vi "Example 02e - Lua Scripts from Lua File.vi"() -> ()   [LabVIEW 2020]
uses:
  Lua for LabVIEW/Lua/Lua.lvclass
panel:
  out "-number":dbl
  out "-integer":i64
  out "!boolean":bool
  out "upper(string)":string
  in  "an_integer":i64=58812
  in  "a boolean":bool=TRUE
  in  "a string":string="my name is ..."
  in  "a double":dbl=2.2
  out "error out":errorcluster
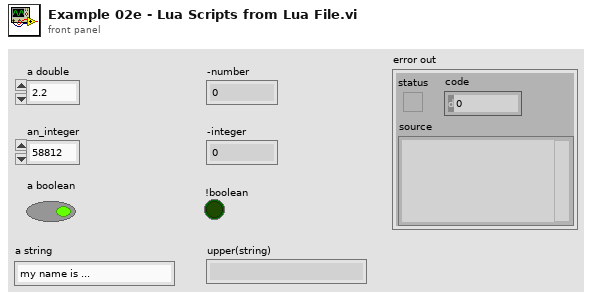
[diagram p1: front panel]
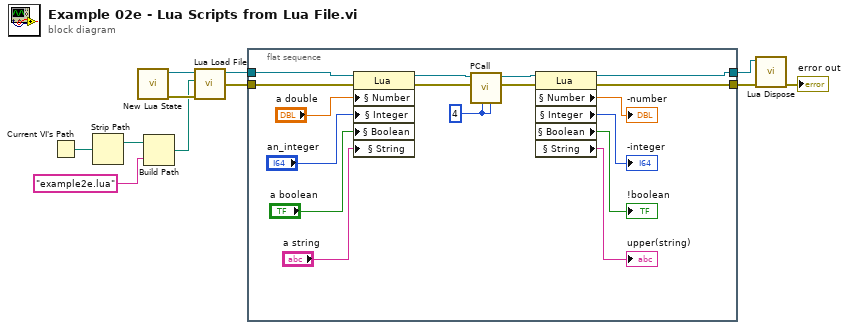
[diagram p0: block diagram]
diagram:
  n1 = Current VI's Path() -> (path=w4:path)
  n2 = Strip Path(path=w4) -> (stripped path=w3:path)  [unwired: 1 out]
  n3 = call "New Lua State.vi"() -> ("error out"=w7:errorcluster, "Lua out"=w8:refnum<class "Lua.lvclass">)  [unwired: 10 in]
  n4 = Build Path(base path=w3, name or relative path="example2e.lua") -> (appended path=w1:path)
  n5 = call "Lua Load File.vi"("error in (no error)"=w7, "filename"=w1, "Lua in"=w8) -> ("error out"=w6:errorcluster, "Lua out"=w5:refnum<class "Lua.lvclass">)  [unwired: 7 in]
  n6 = flat-sequence {
    tunnel: w5 -> [w24]
    tunnel: w6 -> [w23]
    tunnel: [w27] -> w10
    tunnel: [w26] -> w9
    frame #0 {
      w12 = 4 ("nargs")
      n7 = property class="Lua"(reference=w24, error in=w23, "§ Number"="a double", "§ Integer"="an_integer", "§ Boolean"="a boolean", "§ String"="a string") -> (reference out=w25:refnum<class "Lua.lvclass">, error out=w14:errorcluster)
      n8 = call-dynamic "PCall.vi"("nresults"=w12, "nargs"=w12, "error in (no error)"=w14, "Lua in"=w25) -> ("error out"=w13:errorcluster, "Lua out"=w28:refnum<class "Lua.lvclass">)  [unwired: 6 in]
      n9 = property class="Lua"(reference=w28, error in=w13) -> (reference out=w26:refnum<class "Lua.lvclass">, error out=w27:errorcluster, "§ Number"=→"-number":dbl, "§ Integer"=→"-integer":i64, "§ Boolean"=→"!boolean":bool, "§ String"=→"upper(string)":string)
    }
  }
  n10 = call-dynamic "Lua Dispose.vi"("error in (no error)"=w10, "Lua in"=w9) -> ("error out"=→"error out":errorcluster)  [unwired: 9 in]
